vi "UpdateEditors.vi"(8 "error in (no error)":errorcluster, 10 "Array":refnum<vi>[](array[refnum]), 11 "TreeControl in":refnum<vi>) -> (0 "error out":errorcluster)   [LabVIEW 2019, in "ScriptManager.lvlib"]
uses:
  ScriptManager.lvlib
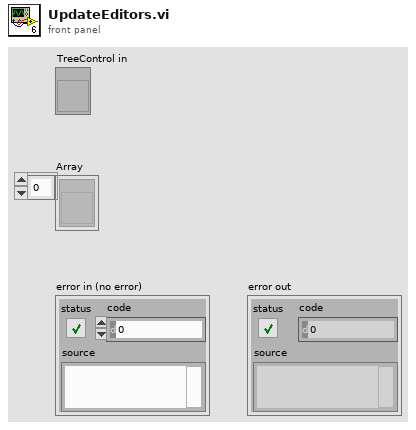
[diagram p1: front panel]
types:
  T1 = enum8{"Enabled", "Disabled", "Disabled and Grayed Out"}
  T2 = enum8{"Enabled", "Disabled", "Disabled and Grayed Out"}[]
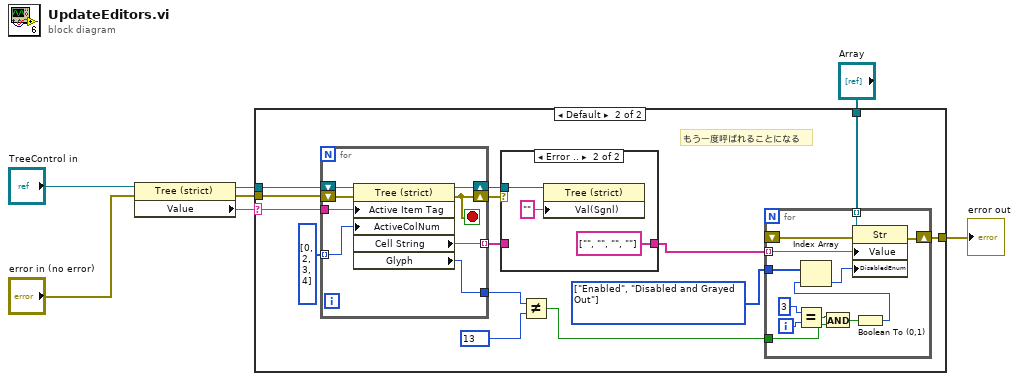
[diagram p0: block diagram]
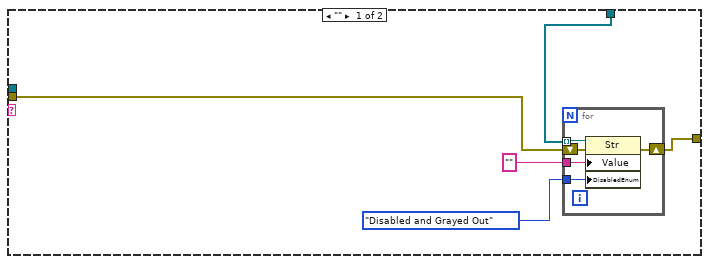
[diagram p2: hidden frame]
diagram:
  n1 = property class="Tree (strict)"(reference="TreeControl in", error in="error in (no error)") -> (reference out=w5:refnum<vi>, error out=w3:errorcluster, "Value"=w4:string)
  n2 = case shown="Default" w4 {
    selector: w4 -> [_ w28]
    tunnel: w5 -> [_ w31]
    tunnel: "Array" -> [w10 w20]
    tunnel: w3 -> [w9 w19]
    tunnel: [w8 w18] -> w2
    frame "" {
      n3 = for {
        tunnel: w10 -> [w17] mode=indexing
        tunnel: T1."Disabled and Grayed Out" ("Disabled") -> [w16]
        tunnel: "" ("Descriptoin") -> [w15]
        shift-right: [w13] -> w8
        shift-left: w9 -> [w14]
        n4 = property on="Property Node" class="Str"(reference=w17, error in=w14, "Value"=w15, "DisabledEnum"=w16) -> (error out=w13:errorcluster)  [unwired: 1 out]
      }
    }
    frame Default {
      w21 = T2 [enum."Enabled", enum."Disabled and Grayed Out"] items=["Enabled", "Disabled", "Disabled and Grayed Out"] ("Disabled")
      # "もう一度呼ばれることになる"
      n5 = for {
        tunnel: w28 -> [w37]
        shift-right: [w38] -> w29
        shift-left: w31 -> [w39]
        shift-right: [w32] -> w30
        shift-left: w19 -> [w36]
        tunnel: [w35] -> w27 mode=indexing
        tunnel: i32[] [0, 2, 3, 4] -> [w34] mode=indexing
        tunnel: [w33] -> w24
        stop <- w32 stop-if-true
        n6 = property class="Tree (strict)"(reference=w39, error in=w36, "Active Item Tag"=w37, "ActiveColNum"=w34) -> (reference out=w38:refnum<vi>, error out=w32:errorcluster, "Cell String"=w35:string, "Glyph"=w33:i32)
      }
      n7 = case shown="Error .." w30 {
        tunnel: w29 -> [_ w55]
        tunnel: w27 -> [w52 _]
        tunnel: [w52 string[] ["", "", "", ""]] -> w26
        frame No Error {
        }
        frame Error {
          n8 = property class="Tree (strict)"(reference=w55, "Val(Sgnl)"="" ("Value")) -> ()  [unwired: 1 in, 2 out]
        }
      }
      n9 = Not Equal?(x=w24, y=13) -> (x != y?=w22:bool)
      n10 = for {
        tunnel: w20 -> [w51] mode=indexing
        tunnel: w26 -> [w50] mode=indexing
        tunnel: w22 -> [w47]
        tunnel: w21 -> [w45]
        shift-right: [w42] -> w18
        shift-left: _ -> [w41]
        i -> [w49]
        n11 = Equal?(x=3, y=w49) -> (x = y?=w48:bool)
        n12 = And(x=w48, y=w47) -> (x .and. y?=w40:bool)
        n13 = Boolean To (0,1)(Boolean=w40) -> (0, 1=w44:i16)
        n14 = Index Array(array=w45, index=w44) -> (element=w43:T1)
        n15 = property on="Property Node" class="Str"(reference=w51, error in=w41, "Value"=w50, "DisabledEnum"=w43) -> (error out=w42:errorcluster)  [unwired: 1 out]
      }
    }
  }
  "error out" <- w2
